vi "Configure.vi"(8 "error in (no error)":errorcluster, 10 "Args":string[](array[string]), 11 "Init in":refnum<class "Init.lvclass">) -> (0 "error out":errorcluster, 3 "Init out":refnum<class "Init.lvclass">)   [LabVIEW 2020, in "Init.lvlib" / "Init.lvclass"]
uses:
  Init.lvclass
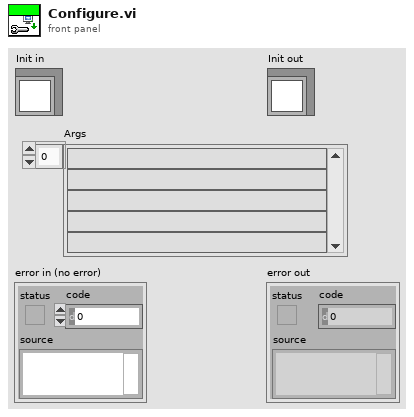
[diagram p1: front panel]
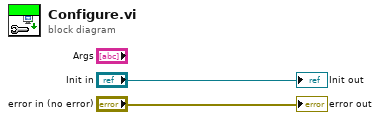
[diagram p0: block diagram]
diagram:
  "error out" <- "error in (no error)"
  "Init out" <- "Init in"
